vi "Identities.vi"(8 "error in (no error)":errorcluster, 11 "VolatusAPI in":refnum<class "VolatusAPI.lvclass">) -> (0 "error out":errorcluster, 2 "Identities":refnum<class "Identity.lvclass">[](array[class]), 3 "VolatusAPI out":refnum<class "VolatusAPI.lvclass">)   [LabVIEW 2020, in "Volatus.lvlib" / "VolatusAPI.lvclass"]
uses:
  VolatusAPI.lvclass
  Identity/Identity.lvclass
  VolatusAPI.lvclass/VolatusAPI.ctl
  ApiIdentity/ApiIdentity.lvclass
  C:/dev/lv20CE/relink/lv-volatus/Volatus/ApiIdentity/ApiIdentity.lvclass
  C:/dev/lv20CE/relink/lv-volatus/Volatus/Identity/Identity.lvclass
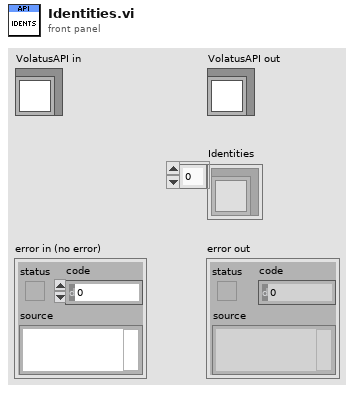
[diagram p1: front panel]
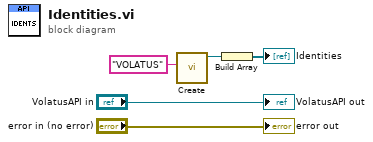
[diagram p0: block diagram]
diagram:
  n1 = call "Create.vi"("API ID"="VOLATUS") -> ("ApiIdentity out"=w3:refnum<class "ApiIdentity.lvclass">)  [unwired: 10 in]
  n2 = Build Array(w3) -> (→"Identities":refnum<class "ApiIdentity.lvclass">[])
  "error out" <- "error in (no error)"
  "VolatusAPI out" <- "VolatusAPI in"
